vi "GetSSMStatusString.vi"(7 "Clear?":bool, 11 "Message":string) -> (3 "Queue Status":string)   [LabVIEW 2018, in "Test.lvclass"]
uses:
  Test.lvclass
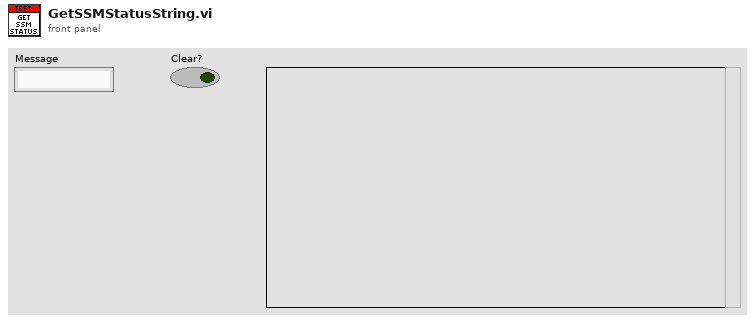
[diagram p1: front panel]
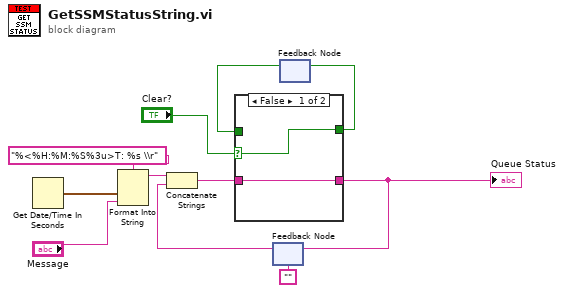
[diagram p0: block diagram]
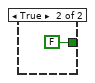
[diagram p2: hidden frame]
diagram:
  n1 = Get Date/Time In Seconds() -> (seconds since 1Jan1904=w1:timestamp)
  n2 = Format Into String(format string="%<%H:%M:%S%3u>T: %s \\r", w1, "Message") -> (resulting string=w9:string)  [unwired: 2 in, 1 out]
  n3 = feedback #1("") -> (w8:string)
  n4 = Concatenate Strings(w9, w8) -> (w6:string)
  n5 = feedback #2() -> (w2:bool)  [unwired: 1 in]
  n6 = case shown="False" "Clear?" {
    selector: "Clear?" -> [w12 _]
    tunnel: w6 -> [w13 _]
    tunnel: [w13 _] -> w5
    tunnel: [w12 FALSE] -> w4
    tunnel: w2 -> [_ _]
    frame False {
    }
    frame True {
    }
  }
  "Queue Status" <- w5
  n7 = feedback-in #1(w5) -> ()
  n8 = feedback-in #2(w4) -> ()
